vi "create fpga resource.vi"(0 "Refnum in":refnum<k20>, 5 "Resource name":string, 7 "Channel FXP type":T1, 9 "Hardware Data type":variant, 11 "error in (no error)":errorcluster) -> (4 "Refnum out":refnum<k20>, 6 "fpga res type":T2, 10 "type supported":bool, 15 "error out":errorcluster)   [LabVIEW 2015, in "io runtime.lvclass"]
uses:
  io runtime.lvclass
  configuration/fpga resource supported data types.ctl
  <vilib>/fxp/LVFixedPointRepBitsTypeDef.ctl
  FXP I_20_5.ctl
  FXP I_24_5.ctl
  FXP I_24_10.ctl
  <vilib>/NI/LVFPGA Adv Session Resources/OpenByNameSubVI.vi
  <vilib>/rvi/interface/common/dynamic/niFpgaEscapeDelimiterAndNull.vi
  <vilib>/Utility/error.llb/Error Cluster From Error Code.vi
  <vilib>/NI/LVFPGA Adv Session Resources/OpenByName.xnode
  configuration/io configuration.lvclass
  <vilib>/NI/LVFPGA Adv Session Resources/LVFPGAAdvSessionResources.lvlib
  <vilib>/Utility/Data Type/NI_Data Type.lvlib
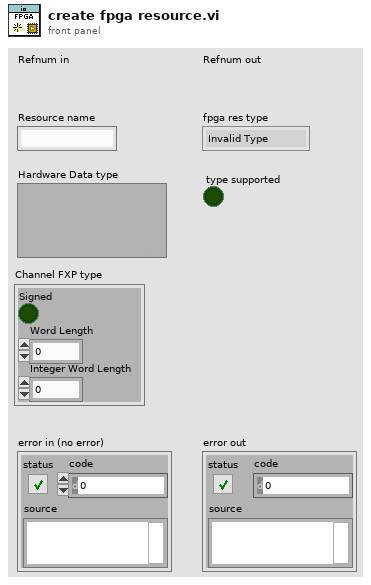
[diagram p1: front panel]
types:
  T1 = typedef "LVFixedPointRepBitsTypeDef.ctl" = cluster{"Signed":bool, "Word Length":u32, "Integer Word Length":i32}
  T2 = typedef "io configuration.lvclass/fpga resource supported data types.ctl" = enum16{"Invalid Type", "Single", "I64", "I32", "I16", "I8", "U64", "U32", "U16", "U8", "Boolean", "FXP I,20,5", "FXP I,24,5", "FXP I,24,10", "Fifo 1023,I16"}
  T3 = typedef "NI_Data Type.lvlib/Data Type.ctl" = enum8{"Invalid Type", "Void", "I8", "I16", "I32", "I64", "U8", "U16", "U32", "U64", "Single Float", "Double Float", "Extended Float", "Single Complex", "Double Complex", "Extended Complex", "Enum U8", "Enum U16", "Enum U32", "Enum U64", "Single Float With Unit", "Double Float With Unit", "Extended Float With Unit", "Single Complex with Unit", "Double Complex with Unit", "Extended Complex with Unit", "Boolean", "String", "Path", "Picture", "Tag", "Array", "Cluster", "Variant", "LV Variant", "Waveform", "Timestamp", "Digital Waveform", "Digital Data", "ExpressData", "Refnum", "External Data", "VI", "Poly VI", "LabVIEW Class Instance", "Fixed Point"}
  T4 = cluster{"Name":string, "Depth":u32, "Write? (Deprecated:Use Implementation)":bool, "Physical Channel":u32, "Base Address":u32, "Data Width":u32, "Data Type":enum32{"Boolean", "I8", "I16", "I32", "I64", "U8", "U16", "U32", "U64", "FXP", "CustomControl", "SGL"}, "FXP Properties":variant, "Write Window Address":u32, "Implementation":enum16{"niFpgaTargetToHost", "niFpgaHostToTarget", "niFpgaPeerToPeerWriter", "niFpgaPeerToPeerReader", "niCoreTargetToHost", "niCoreHostToTarget"}, "Control Set":u32}[]
  T5 = cluster{"Name":string, "type":variant, "indicator?":bool}[]
  T6 = typedef "io runtime.lvclass/FXP I_20_5.ctl" = refnum<k20>
  T7 = typedef "io runtime.lvclass/FXP I_24_5.ctl" = refnum<k20>
  T8 = typedef "io runtime.lvclass/FXP I_24_10.ctl" = refnum<k20>
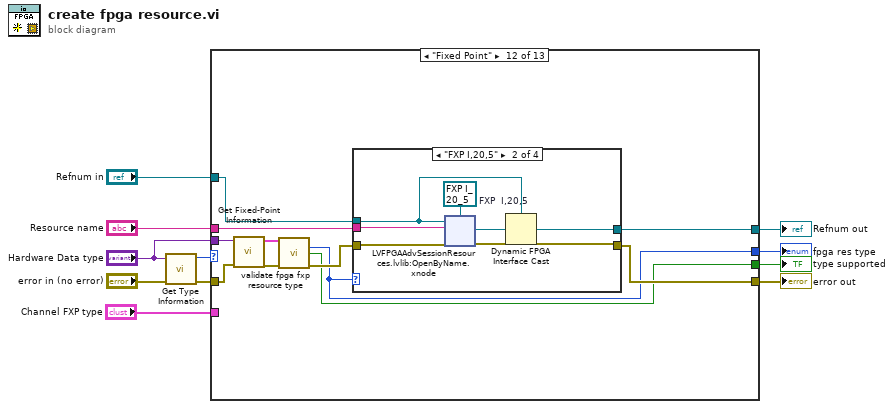
[diagram p0: block diagram]
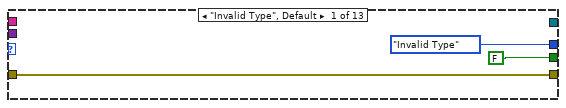
[diagram p2: hidden frame]
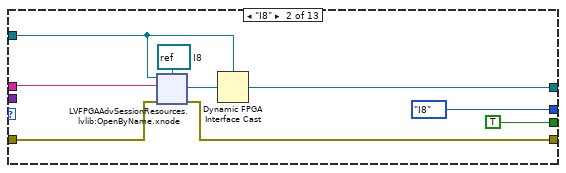
[diagram p3: hidden frame]
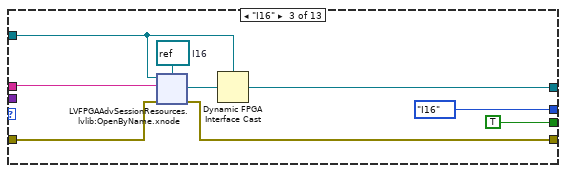
[diagram p4: hidden frame]
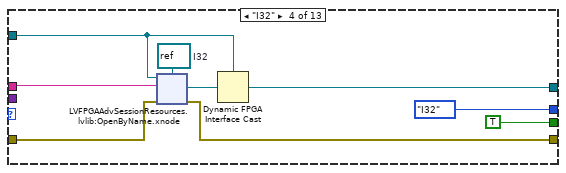
[diagram p5: hidden frame]
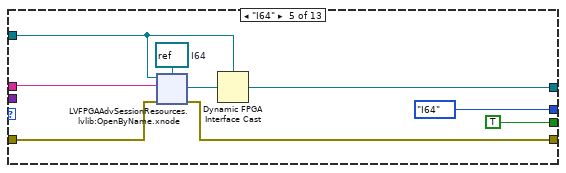
[diagram p6: hidden frame]
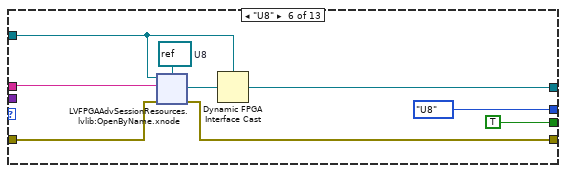
[diagram p7: hidden frame]
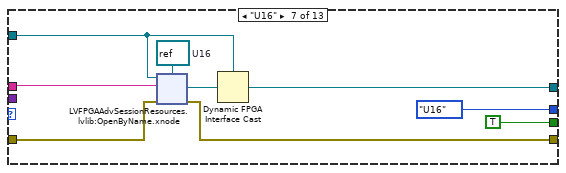
[diagram p8: hidden frame]
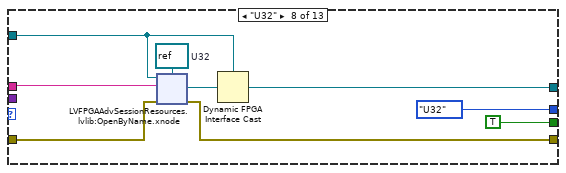
[diagram p9: hidden frame]
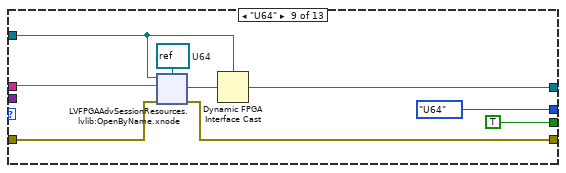
[diagram p10: hidden frame]
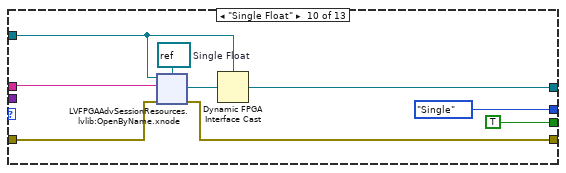
[diagram p11: hidden frame]
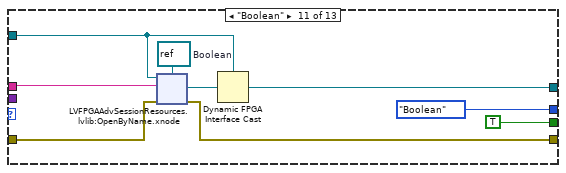
[diagram p12: hidden frame]
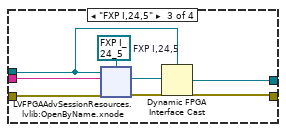
[diagram p14: hidden frame]
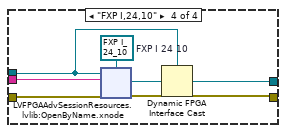
[diagram p15: hidden frame]
diagram:
  n1 = call <vilib>:"Get Type Information.vi"("error in (no error)"="error in (no error)", "Variant"="Hardware Data type") -> ("error out"=w3:errorcluster, "Type"=w2:T3)  [unwired: 5 in, 3 out]
  n2 = case shown="\"Fixed Point\"" w2 {
    tunnel: w3 -> [w13 w15 w43 w65 w87 w109 w131 w153 w175 w197 w219 w244 w307]
    tunnel: [FALSE TRUE TRUE TRUE TRUE TRUE TRUE TRUE TRUE TRUE TRUE w236 _] -> w9
    tunnel: [w13 w20 w42 w64 w86 w108 w130 w152 w174 w196 w218 w239 w307] -> w10
    tunnel: "Hardware Data type" -> [_ _ _ _ _ _ _ _ _ _ _ w245 _]
    tunnel: "Resource name" -> [_ w19 w41 w63 w85 w107 w129 w151 w173 w195 w217 w241 _]
    tunnel: "Refnum in" -> [_ w18 w40 w62 w84 w106 w128 w150 w172 w194 w216 w235 _]
    tunnel: [_ w17 w39 w61 w83 w105 w127 w149 w171 w193 w215 w238 _] -> w8
    tunnel: [fpga_resource_supported_data_types."Invalid Type" ("fpga res type") fpga_resource_supported_data_types."I8" ("fpga res type") fpga_resource_supported_data_types."I16" ("fpga res type") fpga_resource_supported_data_types."I32" ("fpga res type") fpga_resource_supported_data_types."I64" ("fpga res type") fpga_resource_supported_data_types."U8" ("fpga res type") fpga_resource_supported_data_types."U16" ("fpga res type") fpga_resource_supported_data_types."U32" ("fpga res type") fpga_resource_supported_data_types."U64" ("fpga res type") fpga_resource_supported_data_types."Single" ("fpga res type") fpga_resource_supported_data_types."Boolean" ("fpga res type") w237 _] -> w7
    tunnel: "Channel FXP type" -> [_ _ _ _ _ _ _ _ _ _ _ _ _]
    frame "Invalid Type", Default {
    }
    frame "I8" {
      w21 = refnum<k20> refnum  # I8
      n3 = xnode "LVFPGAAdvSessionResources.lvlib:OpenByName.xnode"("FPGA VI Reference in"=w18, "Resource name in"=w19, "Single resource reference type in"=w21, "Error in"=w15) -> ("Single resource reference out"=w22:refnum<k20>, "Error out"=w20:errorcluster)  [unwired: 1 out]
      n4 = Dynamic FPGA Interface Cast(Session In=w18, Type=w22) -> (Session Out=w17:refnum<k20>)
    }
    frame "I16" {
      w37 = refnum<k20> refnum  # I16
      n5 = xnode "LVFPGAAdvSessionResources.lvlib:OpenByName.xnode"("FPGA VI Reference in"=w40, "Resource name in"=w41, "Single resource reference type in"=w37, "Error in"=w43) -> ("Single resource reference out"=w44:refnum<k20>, "Error out"=w42:errorcluster)  [unwired: 1 out]
      n6 = Dynamic FPGA Interface Cast(Session In=w40, Type=w44) -> (Session Out=w39:refnum<k20>)
    }
    frame "I32" {
      w59 = refnum<k20> refnum  # I32
      n7 = xnode "LVFPGAAdvSessionResources.lvlib:OpenByName.xnode"("FPGA VI Reference in"=w62, "Resource name in"=w63, "Single resource reference type in"=w59, "Error in"=w65) -> ("Single resource reference out"=w66:refnum<k20>, "Error out"=w64:errorcluster)  [unwired: 1 out]
      n8 = Dynamic FPGA Interface Cast(Session In=w62, Type=w66) -> (Session Out=w61:refnum<k20>)
    }
    frame "I64" {
      w81 = refnum<k20> refnum  # I64
      n9 = xnode "LVFPGAAdvSessionResources.lvlib:OpenByName.xnode"("FPGA VI Reference in"=w84, "Resource name in"=w85, "Single resource reference type in"=w81, "Error in"=w87) -> ("Single resource reference out"=w88:refnum<k20>, "Error out"=w86:errorcluster)  [unwired: 1 out]
      n10 = Dynamic FPGA Interface Cast(Session In=w84, Type=w88) -> (Session Out=w83:refnum<k20>)
    }
    frame "U8" {
      w103 = refnum<k20> refnum  # U8
      n11 = xnode "LVFPGAAdvSessionResources.lvlib:OpenByName.xnode"("FPGA VI Reference in"=w106, "Resource name in"=w107, "Single resource reference type in"=w103, "Error in"=w109) -> ("Single resource reference out"=w110:refnum<k20>, "Error out"=w108:errorcluster)  [unwired: 1 out]
      n12 = Dynamic FPGA Interface Cast(Session In=w106, Type=w110) -> (Session Out=w105:refnum<k20>)
    }
    frame "U16" {
      w125 = refnum<k20> refnum  # U16
      n13 = xnode "LVFPGAAdvSessionResources.lvlib:OpenByName.xnode"("FPGA VI Reference in"=w128, "Resource name in"=w129, "Single resource reference type in"=w125, "Error in"=w131) -> ("Single resource reference out"=w132:refnum<k20>, "Error out"=w130:errorcluster)  [unwired: 1 out]
      n14 = Dynamic FPGA Interface Cast(Session In=w128, Type=w132) -> (Session Out=w127:refnum<k20>)
    }
    frame "U32" {
      w147 = refnum<k20> refnum  # U32
      n15 = xnode "LVFPGAAdvSessionResources.lvlib:OpenByName.xnode"("FPGA VI Reference in"=w150, "Resource name in"=w151, "Single resource reference type in"=w147, "Error in"=w153) -> ("Single resource reference out"=w154:refnum<k20>, "Error out"=w152:errorcluster)  [unwired: 1 out]
      n16 = Dynamic FPGA Interface Cast(Session In=w150, Type=w154) -> (Session Out=w149:refnum<k20>)
    }
    frame "U64" {
      w169 = refnum<k20> refnum  # U64
      n17 = xnode "LVFPGAAdvSessionResources.lvlib:OpenByName.xnode"("FPGA VI Reference in"=w172, "Resource name in"=w173, "Single resource reference type in"=w169, "Error in"=w175) -> ("Single resource reference out"=w176:refnum<k20>, "Error out"=w174:errorcluster)  [unwired: 1 out]
      n18 = Dynamic FPGA Interface Cast(Session In=w172, Type=w176) -> (Session Out=w171:refnum<k20>)
    }
    frame "Single Float" {
      w191 = refnum<k20> refnum  # Single Float
      n19 = xnode "LVFPGAAdvSessionResources.lvlib:OpenByName.xnode"("FPGA VI Reference in"=w194, "Resource name in"=w195, "Single resource reference type in"=w191, "Error in"=w197) -> ("Single resource reference out"=w198:refnum<k20>, "Error out"=w196:errorcluster)  [unwired: 1 out]
      n20 = Dynamic FPGA Interface Cast(Session In=w194, Type=w198) -> (Session Out=w193:refnum<k20>)
    }
    frame "Boolean" {
      w213 = refnum<k20> refnum  # Boolean
      n21 = xnode "LVFPGAAdvSessionResources.lvlib:OpenByName.xnode"("FPGA VI Reference in"=w216, "Resource name in"=w217, "Single resource reference type in"=w213, "Error in"=w219) -> ("Single resource reference out"=w220:refnum<k20>, "Error out"=w218:errorcluster)  [unwired: 1 out]
      n22 = Dynamic FPGA Interface Cast(Session In=w216, Type=w220) -> (Session Out=w215:refnum<k20>)
    }
    frame "Fixed Point" {
      n23 = call <vilib>:"Get Fixed-Point Information.vi"("error in (no error)"=w244, "Variant"=w245) -> ("error out"=w243:errorcluster, "FXP Representation"=w242:T1)  [unwired: 6 in, 2 out]
      n24 = call "validate fpga fxp resource type.vi"("FXP Representation"=w242, "error in (no error)"=w243) -> ("fpga res type"=w237:T2, "FXP type supported"=w236:bool, "error out"=w240:errorcluster)  [unwired: 11 in]
      n25 = case shown="\"FXP I,20,5\"" w237 {
        tunnel: w235 -> [_ w248 w273 w292]
        tunnel: [_ w252 w272 w291] -> w238
        tunnel: w241 -> [_ w251 w271 w290]
        tunnel: w240 -> [w246 w250 w270 w289]
        tunnel: [w246 w249 w269 w288] -> w239
        frame "Invalid Type", Default {
        }
        frame "FXP I,20,5" {
          w247 = T6 refnum  # FXP  I,20,5
          n26 = xnode "LVFPGAAdvSessionResources.lvlib:OpenByName.xnode"("FPGA VI Reference in"=w248, "Resource name in"=w251, "Single resource reference type in"=w247, "Error in"=w250) -> ("Single resource reference out"=w253:T6, "Error out"=w249:errorcluster)  [unwired: 1 out]
          n27 = Dynamic FPGA Interface Cast(Session In=w248, Type=w253) -> (Session Out=w252:refnum<k20>)
        }
        frame "FXP I,24,5" {
          w267 = T7 refnum  # FXP I,24,5
          n28 = xnode "LVFPGAAdvSessionResources.lvlib:OpenByName.xnode"("FPGA VI Reference in"=w273, "Resource name in"=w271, "Single resource reference type in"=w267, "Error in"=w270) -> ("Single resource reference out"=w268:T7, "Error out"=w269:errorcluster)  [unwired: 1 out]
          n29 = Dynamic FPGA Interface Cast(Session In=w273, Type=w268) -> (Session Out=w272:refnum<k20>)
        }
        frame "FXP I,24,10" {
          w287 = T8 refnum  # FXP I 24 10
          n30 = xnode "LVFPGAAdvSessionResources.lvlib:OpenByName.xnode"("FPGA VI Reference in"=w292, "Resource name in"=w290, "Single resource reference type in"=w287, "Error in"=w289) -> ("Single resource reference out"=w293:T8, "Error out"=w288:errorcluster)  [unwired: 1 out]
          n31 = Dynamic FPGA Interface Cast(Session In=w292, Type=w293) -> (Session Out=w291:refnum<k20>)
        }
      }
    }
    frame "Array" {
    }
  }
  "error out" <- w10
  "type supported" <- w9
  "Refnum out" <- w8
  "fpga res type" <- w7
